vi "Create Process.vi"(6 "Database":T1, 8 "Error In":errorcluster, 9 "Run?":bool=TRUE, 10 "Process Name":string, 11 "CS++DSCManager in":refnum<class "CS++DSCManager.lvclass">) -> (0 "Error Out":errorcluster, 3 "CS++DSCManager out":refnum<class "CS++DSCManager.lvclass">)   [LabVIEW 2016, in "CS++DSCManager.lvlib" / "CS++DSCManager.lvclass"]
doc: "Creates an empty process in the Shared Variable Engine (SVE) on the host computer. The process that you want to create replaces an existing process if the two processes have the same name."
uses:
  CS++DSCManager.lvclass
  <vilib>/lvdsc/NI_DSC.lvlib
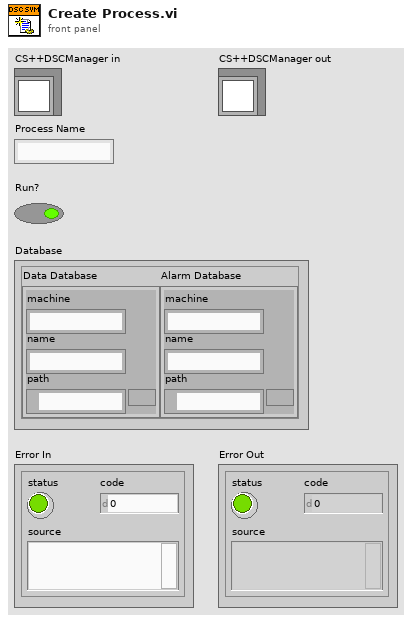
[diagram p1: front panel]
types:
  T1 = cluster{"Data Database":cluster{"machine":string, "name":string, "path":path}, "Alarm Database":cluster{"machine":string, "name":string, "path":path}}
  T2 = cluster{"machine":string, "name":string, "path":path}
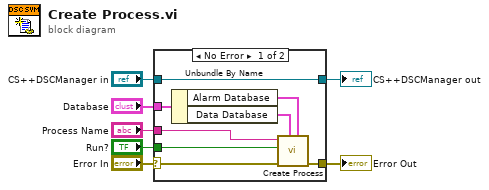
[diagram p0: block diagram]
diagram:
  n1 = case shown="No Error" "Error In" {
    selector: "Error In" -> [w14 w17]
    tunnel: [w13 w17] -> w6
    tunnel: [w15 w16] -> w4
    tunnel: "CS++DSCManager in" -> [w15 w16]
    tunnel: "Run?" -> [w12 _]
    tunnel: "Process Name" -> [w11 _]
    tunnel: "Database" -> [w10 _]
    frame No Error {
      n2 = Unbundle By Name(w10) -> ("Alarm Database"=w8:T2, "Data Database"=w9:T2)
      n3 = call <vilib>:"Create Process.vi"("alarm database"=w8, "data database"=w9, "error in (no error)"=w14, "run?"=w12, "process name"=w11) -> ("error out"=w13:errorcluster)  [unwired: 5 in, 1 out]
    }
    frame Error {
    }
  }
  "Error Out" <- w6
  "CS++DSCManager out" <- w4
